vi "RSZVB Load Mixer Delay Values.vi"(7 "File (\"\")":string, 8 "error in (no error)":errorcluster {"code" format="%.0x"}, 9 "Type":i32(ring) items=["File", "Constant Delay"], 10 "Channel (1)":i32=1, 11 "VISA session":refnum<visa-resource-name>) -> (0 "error out":errorcluster {"code" format="%.0x"}, 3 "dup VISA session":refnum<visa-resource-name>)   [LabVIEW 2011]
doc: "Loads the known delay values of a calibration mixer, to be used as a reference for a mixer delay measurement calibration. Mixer delay measurements are controlled using the SENSe<Ch>:FREQuency:MDELay... commands. \n\nRemote-control command(s):\nMMEMory:LOAD:MDAData <Channel>, '<file_name>' | CDELay"
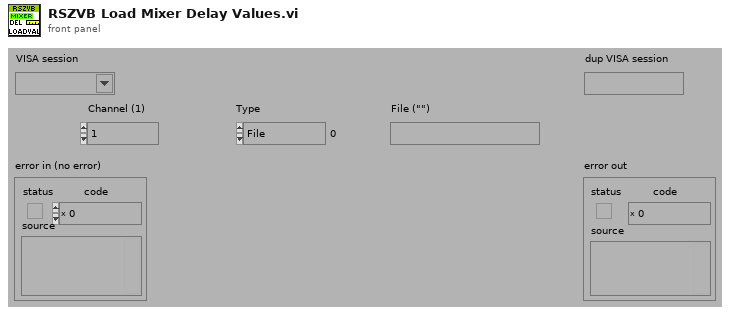
[diagram p1: front panel]
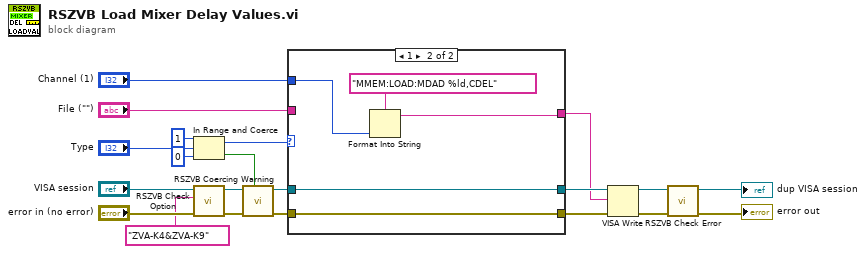
[diagram p0: block diagram]
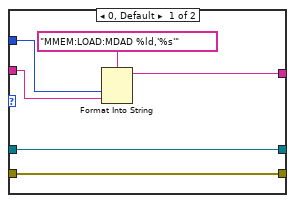
[diagram p2: hidden frame]
diagram:
  n1 = In Range and Coerce(upper limit=1, x="Type", lower limit=0) -> (coerced(x)=w15:i32, In Range?=w12:bool)
  n2 = call "RSZVB Check Option.vi"("error in (no error)"="error in (no error)", "Options"="ZVA-K4&ZVA-K9", "VISA session"="VISA session") -> ("error out"=w14:errorcluster, "dup VISA session"=w13:refnum<visa-resource-name>)  [unwired: 7 in]
  n3 = call "RSZVB Coercing Warning.vi"("In Range?"=w12, "error in (no error)"=w14, "VISA session"=w13) -> ("error out"=w11:errorcluster, "dup VISA session"=w10:refnum<visa-resource-name>)  [unwired: 7 in]
  n4 = case shown="1" w15 {
    tunnel: w11 -> [w22 w31]
    tunnel: w10 -> [w23 w32]
    tunnel: [w23 w32] -> w6
    tunnel: [w22 w31] -> w7
    tunnel: "Channel (1)" -> [w26 w28]
    tunnel: "File (\"\")" -> [w25 _]
    tunnel: [w24 w29] -> w5
    frame 0, Default {
      n5 = Format Into String(format string="MMEM:LOAD:MDAD %ld,'%s'", w26, w25) -> (resulting string=w24:string)  [unwired: 2 in, 1 out]
    }
    frame 1 {
      n6 = Format Into String(format string="MMEM:LOAD:MDAD %ld,CDEL", w28) -> (resulting string=w29:string)  [unwired: 2 in, 1 out]
    }
  }
  n7 = VISA Write(VISA resource name=w6, write buffer=w5, error in (no error)=w7) -> (VISA resource name out=w2:refnum<visa-resource-name>, error out=w4:errorcluster)  [unwired: 1 out]
  n8 = call "RSZVB Check Error.vi"("error in (no error)"=w4, "VISA session"=w2) -> ("error out"=→"error out":errorcluster, "dup VISA session"=→"dup VISA session":refnum<visa-resource-name>)  [unwired: 8 in]
